vi "Find Max Linearity.vi"(8 "error in (no error)":errorcluster, 11 "Linearity Results":T1[](array[typedef])) -> (0 "error out":errorcluster, 3 "Max Linearity %FS":dbl)   [LabVIEW 2026, in "Analysis.lvlib"]
uses:
  Analysis.lvlib
  Linearity Result.ctl
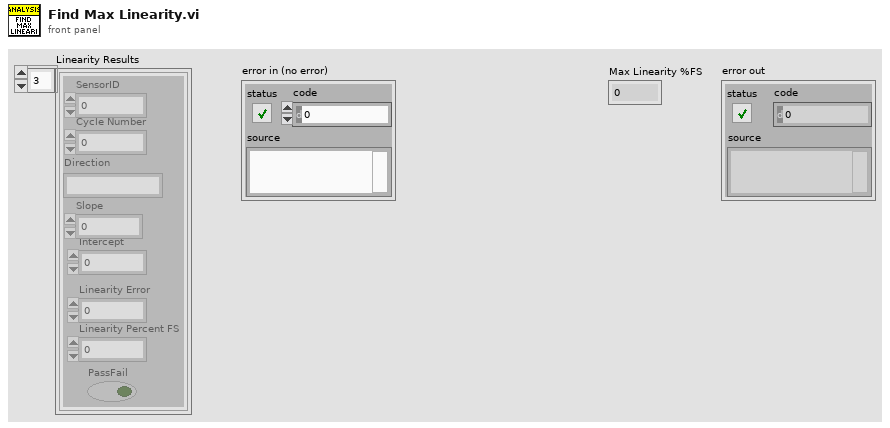
[diagram p1: front panel]
types:
  T1 = typedef "Analysis.lvlib/Linearity Result.ctl" = cluster{"Slope":dbl, "Intercept":dbl, "Cycle Number":i32, "SensorID":i32, "Linearity Error":dbl, "Linearity Percent FS":dbl, "Direction":string, "PassFail":bool}
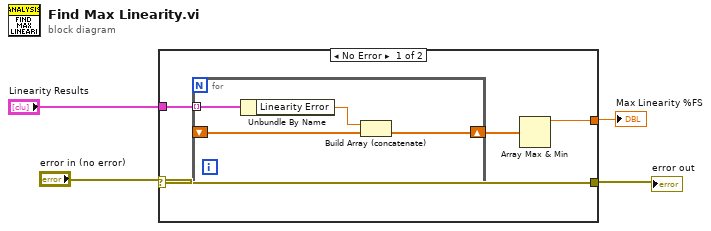
[diagram p0: block diagram]
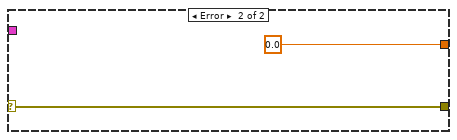
[diagram p2: hidden frame]
diagram:
  n1 = case shown="No Error" "error in (no error)" {
    selector: "error in (no error)" -> [w5 w13]
    tunnel: "Linearity Results" -> [w8 _]
    tunnel: [w6 0.0] -> w3
    tunnel: [w5 w13] -> w2
    frame No Error {
      n2 = for {
        tunnel: w8 -> [w12] mode=indexing
        shift-right: [w10] -> w7
        shift-left: _ -> [w9]
        n3 = Unbundle By Name(w12) -> ("Linearity Error"=w11:dbl)
        n4 = Build Array (concatenate)(w11, w9) -> (w10:dbl[])
      }
      n5 = Array Max & Min(array=w7) -> (max value=w6:dbl)  [unwired: 3 out]
    }
    frame Error {
    }
  }
  "error out" <- w2
  "Max Linearity %FS" <- w3
